vi "MGI Init Daemon.vi"(10 "Err Dir":path, 11 "MGI Error Reporter Base In":refnum<class "MGI Error Reporter Base.lvclass">) -> (0 "Custom User Event":refnum<user-event>, 1 "Handler User Event":refnum<user-event>, 3 "MGI Error Reporter Base Out":refnum<class "MGI Error Reporter Base.lvclass">)   [LabVIEW 2020, in "MGI Error Reporter Base.lvclass"]
doc: "Creates the Error Queue and User Events used by the MGI Error Reporter Base VIs. This VI must be called for the MGI Error Reporter Base VIs to work.\n\nAuthored by Shawn Walpole\nsupport@mooregoodideas.com\nwww.mooregoodideas.com\n\nCopyright (c) 2013, Moore Good Ideas, Inc.\n\nAll rights reserved.\n\nRedistribution and use in source and binary forms, with or without modification, are permitted provided that the following conditions are met:\n\n * Redistributions of source code must retain the above copyright notice, this list of conditions and the following disclaimer.\n * Redistributions in binary form must reproduce the above copyright notice, this list of conditions and the following disclaimer in the documentation and/or other materials provided with the distribution.\n * Neither the name of Moore Good Ideas, Inc. nor the names of its contributors may be used to endorse or promote products derived from this software without specific prior written permission.\n\nTHIS SOFTWARE IS PROVIDED BY THE COPYRIGHT HOLDERS AND CONTRIBUTORS \"AS IS\" AND ANY EXPRESS OR IMPLIED WARRANTIES, INCLUDING, BUT NOT LIMITED TO, THE IMPLIED WARRANTIES OF MERCHANTABILITY AND FITNESS FOR A PARTICULAR PURPOSE ARE DISCLAIMED. IN NO EVENT SHALL THE COPYRIGHT OWNER OR CONTRIBUTORS BE LIABLE FOR ANY DIRECT, INDIRECT, INCIDENTAL, SPECIAL, EXEMPLARY, OR CONSEQUENTIAL DAMAGES (INCLUDING, BUT NOT LIMITED TO, PROCUREMENT OF SUBSTITUTE GOODS OR SERVICES; LOSS OF USE, DATA, OR PROFITS; OR BUSINESS INTERRUPTION) HOWEVER CAUSED AND ON ANY THEORY OF LIABILITY, WHETHER IN CONTRACT, STRICT LIABILITY, OR TORT (INCLUDING NEGLIGENCE OR OTHERWISE) ARISING IN ANY WAY OUT OF THE USE OF THIS SOFTWARE, EVEN IF ADVISED OF THE POSSIBILITY OF SUCH DAMAGE."
uses:
  <userlib>/_MGI/Error Reporter/MGI Error Reporter Base/MGI Error Reporter Base.lvclass
  <userlib>/_MGI/Error Reporter/MGI Error Reporter Base/Protected/MGI Cmd Enum.ctl
  <userlib>/_MGI/Error Reporter/MGI Error Reporter Base/MGI Error Reporter Base.lvclass/MGI Error Reporter Base.ctl
  <userlib>/_MGI/Error Reporter/MGI Error Reporter Base/Private/MGI Globals.vi
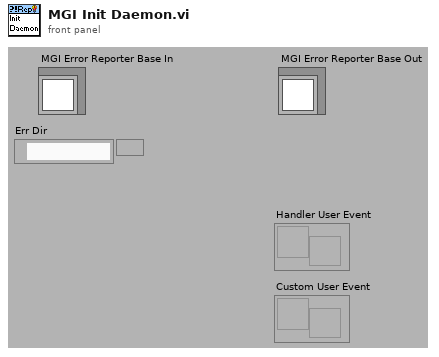
[diagram p1: front panel]
types:
  T1 = typedef "MGI Error Reporter Base.lvclass/MGI Cmd Enum.ctl" = enum16{"Quit", "Show UI"}
  T2 = cluster{"read mode":enum16{"polling", "blocking"}, "write mode":enum16{"polling", "blocking"}}
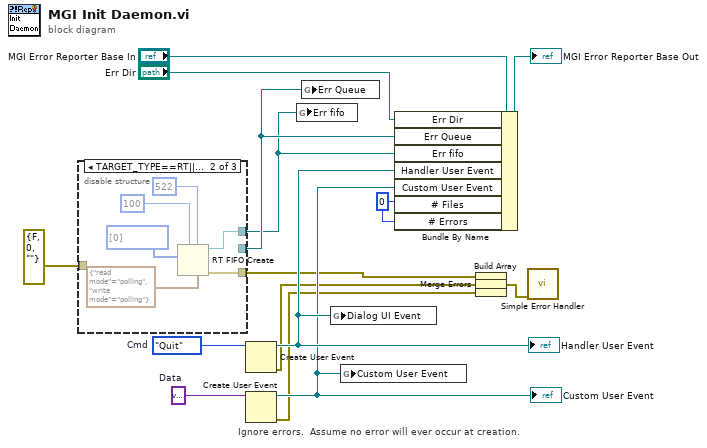
[diagram p0: block diagram]
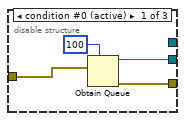
[diagram p2: hidden frame]
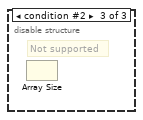
[diagram p3: hidden frame]
diagram:
  w8 = 0 ("# Files")
  w14 = variant  # Data
  w15 = MGI_Cmd_Enum."Quit"  # Cmd
  # "Ignore errors.  Assume no error will ever occur at creation."
  n1 = disable-structure shown="TARGET_TYPE==RT||TARGET_TYPE==Embedded" {
    disable-tunnel: errorcluster {"status"=FALSE, "code"=0, "source"=""} ("error") -> [w20 _ _]
    disable-tunnel: [w18 _ _] -> w11
    disable-tunnel: [_ w23 _] -> w7
    disable-tunnel: [w17 w21 _] -> w4
    frame condition #0 (active) {
      n2 = Obtain Queue(max queue size (-1, unlimited)=100, element data type=w20) -> (queue out=w18:refnum<queue>, error out=w17:errorcluster)  [unwired: 2 in, 2 out]
    }
    frame condition #1 {
      n3 = RT FIFO Create(1:u8[] [0], 4:u32 100 ("size (10)"), 6:u32 522 ("elements in array (1)"), 7:T2 {"read mode"=enum."polling", "write mode"=enum."polling"} ("r/w modes (polling,polling)")) -> (8:w23:refnum<k33>, 11:w21:errorcluster)  [unwired: 4 in, 1 out]
    }
    frame condition #2 {
      # "Not supported"
      n4 = Array Size() -> ()  [unwired: 1 in, 1 out]
    }
  }
  n5 = Create User Event(user event datatype=w15) -> (user event=w10:refnum<user-event>, error out=w2:errorcluster)  [unwired: 1 in]
  "Handler User Event" <- w10
  n6 = Create User Event(user event datatype=w14) -> (user event=w9:refnum<user-event>, error out=w3:errorcluster)  [unwired: 1 in]
  "Custom User Event" <- w9
  n7 = global write "MGI Globals.vi" "Err fifo"(w7) -> ()
  n8 = global write "MGI Globals.vi" "Err Queue"(w11) -> ()
  n9 = global write "MGI Globals.vi" "Dialog UI Event"(w10) -> ()
  n10 = global write "MGI Globals.vi" "Custom User Event"(w9) -> ()
  n11 = Bundle By Name(cluster="MGI Error Reporter Base In", "Err Dir"="Err Dir", "Err Queue"=w11, "Err fifo"=w7, "Handler User Event"=w10, "Custom User Event"=w9, "# Files"=w8, "# Errors"=w8) -> (→"MGI Error Reporter Base Out":refnum<class "MGI Error Reporter Base.lvclass">)
  n12 = Build Array(w4, w2, w3) -> (w1:errorcluster[])
  n13 = Merge Errors(w1) -> (w5:errorcluster)
  n14 = call <vilib>:"Simple Error Handler.vi"("error in (no error)"=w5) -> ()  [unwired: 1 in, 8 out]
